vi "Clear Notification Map.vi"(8 "error in (no error)":errorcluster, 11 "TwinCAT ADS in":refnum<class "TwinCAT ADS.lvclass">) -> (0 "error out":errorcluster, 1 "[Value]":T1[](array[typedef]), 2 "[Symbol Name]":string[](array[string]), 3 "TwinCAT ADS out":refnum<class "TwinCAT ADS.lvclass">, 5 "[Alias]":string[](array[string]))   [LabVIEW 2018, in "TwinCAT ADS.lvclass"]
uses:
  TwinCAT ADS.lvclass
  Controls/Notifcation Map Value.ctl
  TwinCAT ADS.lvclass/TwinCAT ADS.ctl
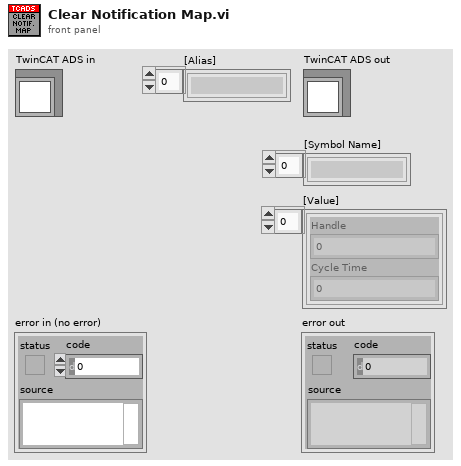
[diagram p1: front panel]
types:
  T1 = typedef "TwinCAT ADS.lvclass/Notifcation Map Value.ctl" = cluster{"Handle":i32, "Cycle Time":i32}
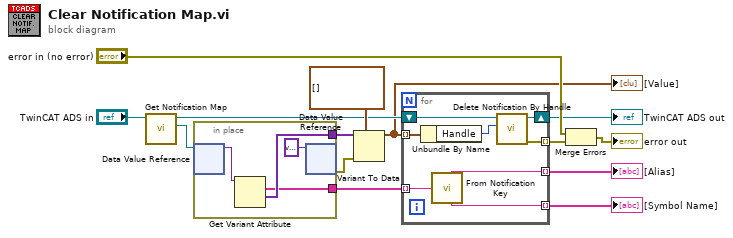
[diagram p0: block diagram]
diagram:
  n1 = call "Get Notification Map.vi"("TwinCAT ADS in"="TwinCAT ADS in") -> ("Notification Map"=w5:refnum<data-value>, "TwinCAT ADS out"=w6:refnum<class "TwinCAT ADS.lvclass">)  [unwired: 8 in, 1 out]
  n2 = in-place {
    in-place-border: [w16] -> w12
    in-place-border: [w15] -> w3
    n3 = in-place-dvr #1(w5) -> (w17:variant)  [unwired: 1 out]
    n4 = Get Variant Attribute(Variant=w17) -> (names=w15:string[], values=w16:variant[])  [unwired: 3 in, 2 out]
    n5 = in-place-dvr #1(variant ("data value")) -> (w13:errorcluster)  [unwired: 1 out]
  }
  n6 = Variant To Data(error in=w13, type=T1[] [], Variant=w12) -> (data=w4:T1[])  [unwired: 1 out]
  "[Value]" <- w4
  n7 = for {
    tunnel: w4 -> [w23] mode=indexing
    shift-right: [w25] -> w10
    shift-left: w6 -> [w26]
    tunnel: [w24] -> w9 mode=indexing
    tunnel: w3 -> [w21] mode=indexing
    tunnel: [w20] -> w2 mode=indexing
    tunnel: [w19] -> w1 mode=indexing
    n8 = Unbundle By Name(w23) -> ("Handle"=w22:i32)
    n9 = call "From Notification Key.vi"("Key"=w21) -> ("Alias"=w20:string, "Symbol Name"=w19:string)  [unwired: 7 in]
    n10 = call "Delete Notification By Handle.vi"("Handle"=w22, "TwinCAT ADS in"=w26) -> ("error out"=w24:errorcluster, "TwinCAT ADS out"=w25:refnum<class "TwinCAT ADS.lvclass">)  [unwired: 8 in]
  }
  "TwinCAT ADS out" <- w10
  "[Symbol Name]" <- w1
  "[Alias]" <- w2
  n11 = Merge Errors("error in (no error)", w9) -> (→"error out":errorcluster)
